vi "BuildSlaveRWr.vi"() -> (0 "RWr":i16[][](array[numeric]))   [LabVIEW 2018]
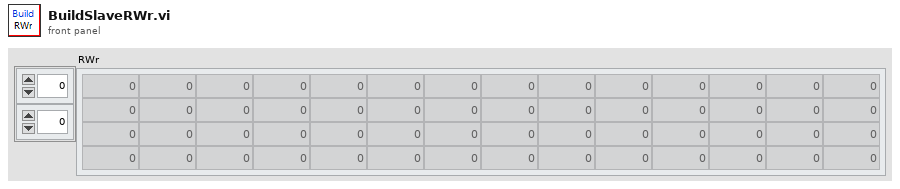
[diagram p1: front panel]
types:
  T1 = cluster{"轮盘预压力":sgl, "泄漏量上限":sgl, "压力上限":sgl, "压力下限":sgl, "风门闭电压上限":sgl, "风门闭电压下限":sgl, "风门开电压上限":sgl, "风门开电压下限":sgl, "LED电流上限":sgl, "LED电流下限":sgl, "气压稳定时间":sgl, "伺服速度":sgl, "INV初始频率":sgl, "INV变化周期":sgl, "INV慢速变化量":sgl, "INV快速变化量":sgl}
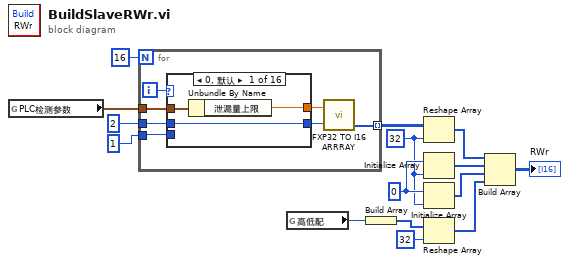
[diagram p0: block diagram]
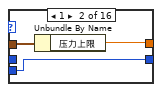
[diagram p2: hidden frame]
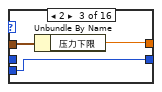
[diagram p3: hidden frame]
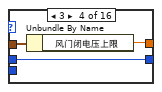
[diagram p4: hidden frame]
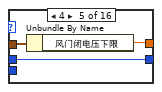
[diagram p5: hidden frame]
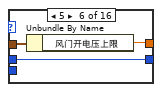
[diagram p6: hidden frame]
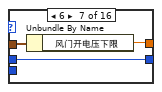
[diagram p7: hidden frame]
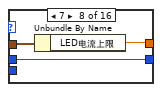
[diagram p8: hidden frame]
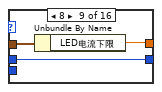
[diagram p9: hidden frame]
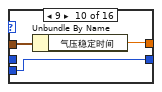
[diagram p10: hidden frame]
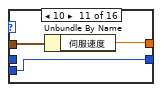
[diagram p11: hidden frame]
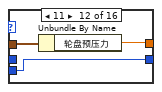
[diagram p12: hidden frame]
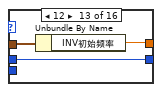
[diagram p13: hidden frame]
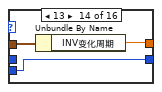
[diagram p14: hidden frame]
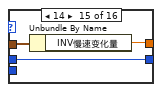
[diagram p15: hidden frame]
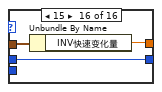
[diagram p16: hidden frame]
diagram:
  w10 = i16 0
  w9 = 32 ("维数大小")
  n1 = global read "全局 1.vi" "PLC检测参数"() -> (w15:T1)
  n2 = for {
    N: 16 -> [_]
    tunnel: w15 -> [w22]
    tunnel: 2 ("位数(2)") -> [w21]
    tunnel: [w17] -> w11 mode=indexing
    tunnel: 1 ("位数(2)") -> [w16]
    i -> [w20]
    n3 = case shown="0, 默认" w20 {
      tunnel: w22 -> [w25 w28 w31 w34 w37 w40 w43 w46 w49 w52 w55 w58 w61 w64 w67 w70]
      tunnel: w21 -> [w23 _ _ w32 w35 w38 w41 w44 w47 _ _ _ w59 _ w65 w68]
      tunnel: [w24 w27 w30 w33 w36 w39 w42 w45 w48 w51 w54 w57 w60 w63 w66 w69] -> w19
      tunnel: [w23 w26 w29 w32 w35 w38 w41 w44 w47 w50 w53 w56 w59 w62 w65 w68] -> w18
      tunnel: w16 -> [_ w26 w29 _ _ _ _ _ _ w50 w53 w56 _ w62 _ _]
      frame 0, Default {
        n4 = Unbundle By Name(w25) -> ("泄漏量上限"=w24:sgl)
      }
      frame 1 {
        n5 = Unbundle By Name(w28) -> ("压力上限"=w27:sgl)
      }
      frame 2 {
        n6 = Unbundle By Name(w31) -> ("压力下限"=w30:sgl)
      }
      frame 3 {
        n7 = Unbundle By Name(w34) -> ("风门闭电压上限"=w33:sgl)
      }
      frame 4 {
        n8 = Unbundle By Name(w37) -> ("风门闭电压下限"=w36:sgl)
      }
      frame 5 {
        n9 = Unbundle By Name(w40) -> ("风门开电压上限"=w39:sgl)
      }
      frame 6 {
        n10 = Unbundle By Name(w43) -> ("风门开电压下限"=w42:sgl)
      }
      frame 7 {
        n11 = Unbundle By Name(w46) -> ("LED电流上限"=w45:sgl)
      }
      frame 8 {
        n12 = Unbundle By Name(w49) -> ("LED电流下限"=w48:sgl)
      }
      frame 9 {
        n13 = Unbundle By Name(w52) -> ("气压稳定时间"=w51:sgl)
      }
      frame 10 {
        n14 = Unbundle By Name(w55) -> ("伺服速度"=w54:sgl)
      }
      frame 11 {
        n15 = Unbundle By Name(w58) -> ("轮盘预压力"=w57:sgl)
      }
      frame 12 {
        n16 = Unbundle By Name(w61) -> ("INV初始频率"=w60:sgl)
      }
      frame 13 {
        n17 = Unbundle By Name(w64) -> ("INV变化周期"=w63:sgl)
      }
      frame 14 {
        n18 = Unbundle By Name(w67) -> ("INV慢速变化量"=w66:sgl)
      }
      frame 15 {
        n19 = Unbundle By Name(w70) -> ("INV快速变化量"=w69:sgl)
      }
    }
    n20 = call "FXP32 TO I16 ARRRAY.vi"("FXP32in"=w19, "位数(2)"=w18) -> ("out I16 array"=w17:i16[])  [unwired: 2 out]
  }
  n21 = global read "全局 1.vi" "高低配"() -> (w8:i16)
  n22 = Build Array(w8) -> (w7:i16[])
  n23 = Reshape Array ("重排数组维数")(w11, w9) -> (w3:i16[])
  n24 = Initialize Array(w10, w9) -> (w2:i16[])
  n25 = Initialize Array(w10, w9) -> (w1:i16[])
  n26 = Reshape Array(w7, 32 ("维数大小")) -> (w5:i16[])
  n27 = Build Array(w3, w2, w1, w5) -> (→"RWr":i16[][])
